vi "Check Protection.vi"(8 "error in (no error)":errorcluster, 10 "String in":string, 11 "Protection in":refnum<class "Protection.lvclass">) -> (0 "error out":errorcluster, 1 "Protection Error":errorcluster, 2 "String out":string, 3 "Protection out":refnum<class "Protection.lvclass">)   [LabVIEW 2013, in "Protections.lvlib" / "Protection.lvclass"]
uses:
  Protection.lvclass
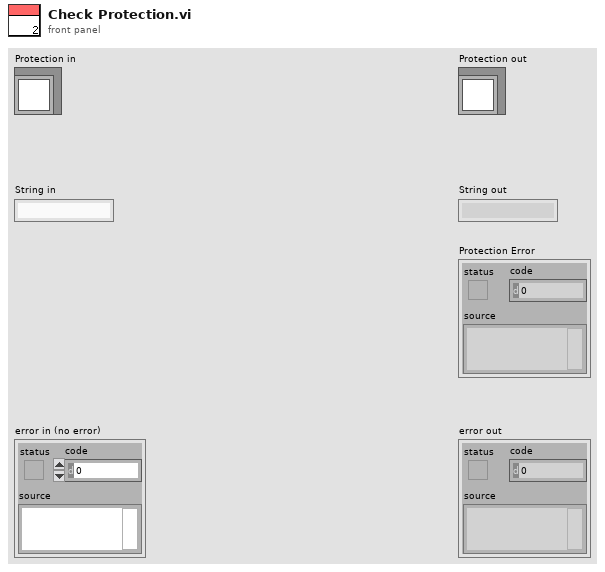
[diagram p1: front panel]
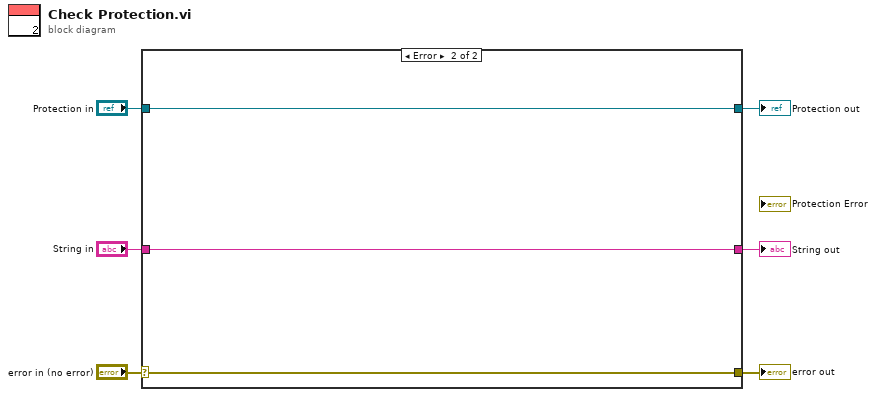
[diagram p0: block diagram]
diagram:
  n1 = case shown="Error" "error in (no error)" {
    selector: "error in (no error)" -> [w8 w12]
    tunnel: [w8 w12] -> w5
    tunnel: [w9 w11] -> w3
    tunnel: "Protection in" -> [w9 w11]
    tunnel: [w7 w10] -> w2
    tunnel: "String in" -> [w7 w10]
    frame No Error {
      # "Wire the error cluster across even in the \"No Error\"\ncase so that warnings get propagated."
    }
    frame Error {
    }
  }
  "error out" <- w5
  "Protection out" <- w3
  "String out" <- w2
